vi "Close RT Queue.vi"(8 "error in":errorcluster, 11 "queue":T2) -> (0 "error out":errorcluster)   [LabVIEW 2022 SP3]
uses:
  RT Controls/RT All Queue.ctl
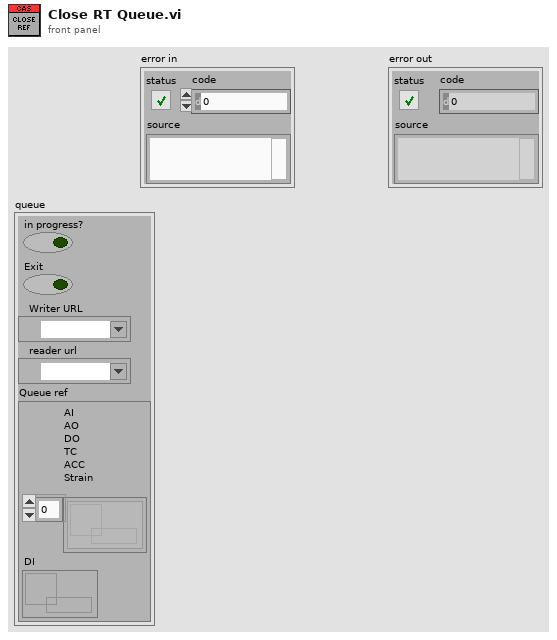
[diagram p1: front panel]
types:
  T1 = typedef "RT All Queue.ctl" = cluster{"AI\nAO\nDO\nTC\nACC\nStrain":refnum<queue>[], "DI":refnum<queue>}
  T2 = cluster{"in progress?":bool, "Exit":bool, "Writer URL":refnum<k21>, "reader url":refnum<k21>, "Queue ref":T1}
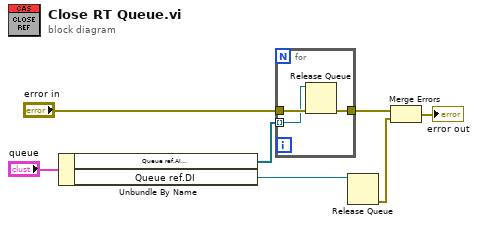
[diagram p0: block diagram]
diagram:
  n1 = Unbundle By Name("queue") -> ("Queue ref.AI\nAO\nDO\nTC\nACC\nStrain"=w5:refnum<queue>[], "Queue ref.DI"=w4:refnum<queue>)
  n2 = for {
    tunnel: "error in" -> [w10]
    tunnel: w5 -> [w9] mode=indexing
    tunnel: [w8] -> w1
    n3 = Release Queue(queue=w9, error in (no error)=w10) -> (error out=w8:errorcluster)  [unwired: 1 in, 2 out]
  }
  n4 = Release Queue(queue=w4) -> (error out=w2:errorcluster)  [unwired: 2 in, 2 out]
  n5 = Merge Errors(w1, w2) -> (→"error out":errorcluster)
